vi "uc480_SetPixelclock.vi"(0 ".NET (Reference)":refnum<k24>, 7 "Pixel clock":i32, 11 "Error In":errorcluster) -> (15 "Error out":errorcluster caption="Error Out")   [LabVIEW 2021]
uses:
  C:/Program Files/Thorlabs/Scientific Imaging/ThorCam/uc480DotNet.dll
  Program Files/Thorlabs/Scientific Imaging/ThorCam/uc480DotNet.dll
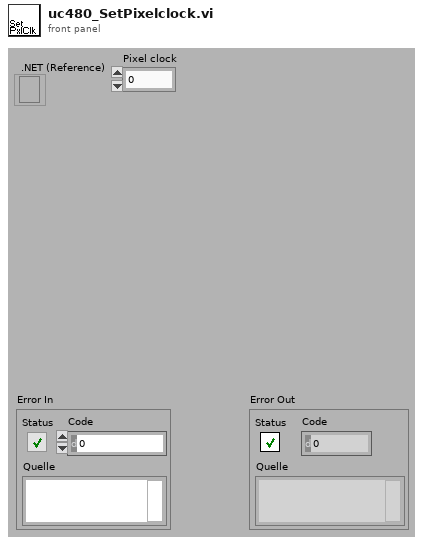
[diagram p1: front panel]
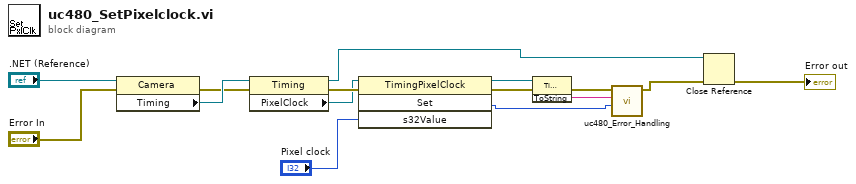
[diagram p0: block diagram]
diagram:
  n1 = property class="Camera"(reference=".NET (Reference)", error in="Error In") -> (error out=w14:errorcluster, "Timing"=w15:refnum<k24>)  [unwired: 1 out]
  n2 = property class="Timing"(reference=w15, error in=w14) -> (reference out=w8:refnum<k24>, error out=w13:errorcluster, "PixelClock"=w12:refnum<k24>)
  n3 = invoke class="TimingPixelClock" method="Set"(reference=w12, error in=w13, "s32Value"="Pixel clock") -> (reference out=w7:refnum<k24>, error out=w6:errorcluster, "Set"=w3:i32)  [unwired: 1 in, 1 out]
  n4 = invoke class="TimingPixelClock" method="ToString"(reference=w7, error in=w6) -> (error out=w5:errorcluster, "ToString"=w4:string)  [unwired: 1 in, 1 out]
  n5 = call "uc480_Error_Handling.vi"("Error Code"=w3, "Error String"=w4, "Error In"=w5) -> ("Error Out"=w2:errorcluster)  [unwired: 8 in]
  n6 = Close Reference(reference=w8, error in (no error)=w2) -> (error out=→"Error out":errorcluster)
